vi "Import_Source_Item_Code.vi"(8 "CONTROL Control":enum32{"IMPRORT", "ADD"}(tab), 9 "UPDATE ONLY":bool, 10 "ITEM_DATA":T2, 11 "connection reference":T1) -> ()   [LabVIEW 2015]
uses:
  <vilib>/addons/database/Connection.llb/Conn ObjectReference.ctl
  Controls/ITEM_INFORMATION_CLUSTER.ctl
  <vilib>/addons/database/Connection.llb/Conn Execute.vi
  <vilib>/addons/database/Recordset.llb/Rec Destroy - Connection.vi
  <vilib>/addons/database/_DB Variant To Data/Database Variant To Data.xnode
  <vilib>/addons/database/NI_Database_API.lvlib
  <vilib>/addons/database/Connection.llb/DB Tools Open Connec (String).vi
panel:
  out "UPDATE ONLY 2":bool
  in  "ADD Button":bool
  in  "EXIT_BUTTON":bool
  out "OK":i32
  out "ERROR":i32
  out "Table":string[][](table)
  in  "IMPORT (*.xlsx)":path
  out "TOTAL":i32
  in  "SHEET":i32
  # "ADD ITEM DATA"
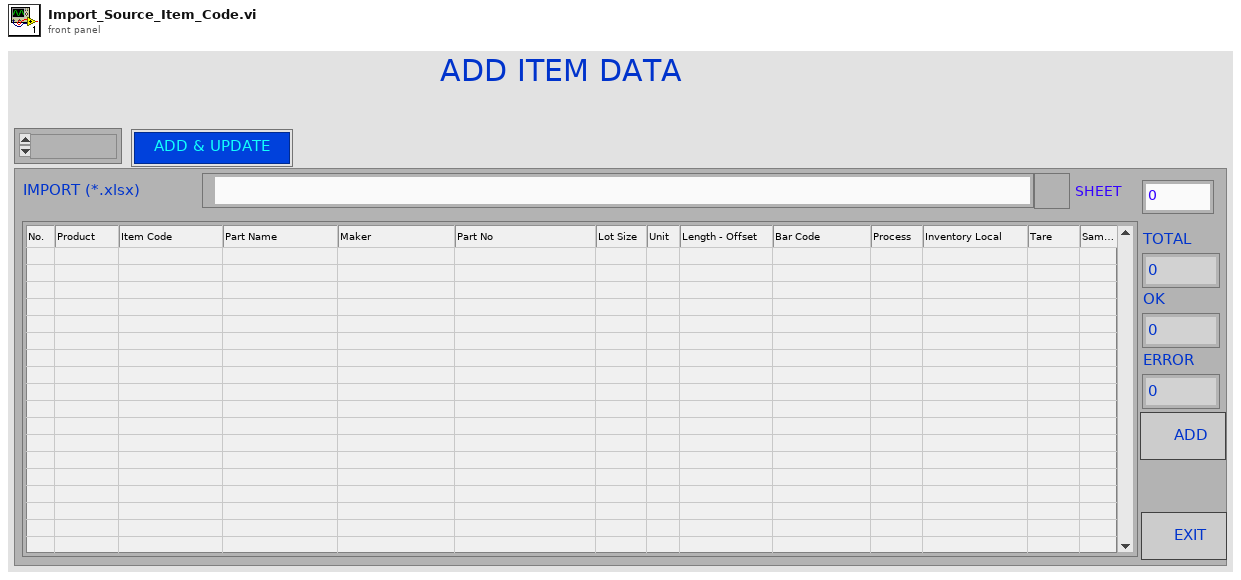
[diagram p1: front panel]
types:
  T1 = typedef "NI_Database_API.lvlib/Conn ObjectReference.ctl" = refnum<k1>
  T2 = cluster{"PRODUCT":string, "ITEM CODE":string, "PART NAME":string, "MAKER":string, "PART NO":string, "LOT SIZE":dbl, "UNIT":string, "LENGTH-OFFSET":string, "BARCODE":string, "PROCESS":string, "INVENTORY LOCAL":string, "TARE":dbl, "SAMPLE":dbl}
  T3 = typedef "ITEM_INFORMATION_CLUSTER.ctl" = cluster{"PRODUCT":string, "ITEM_CODE":string, "PART_NAME":string, "MAKER":string, "PART_NO":string, "LOT_SIZE":dbl, "UNIT":string, "LENGTH-OFFSET":string, "BARCODE":string, "PROCESS":string, "INVENTORY_LOCAL":string, "TARE":dbl, "SAMPLE":dbl}
  T4 = cluster{"PRODUCT":string, "ITEM_CODE":string, "PART_NAME":string, "MAKER":string, "PART_NO":string, "LOT_SIZE":dbl, "UNIT":string, "LENGTH-OFFSET":string, "BARCODE":string, "PROCESS":string, "INVENTORY_LOCAL":string, "TARE":dbl, "SAMPLE":dbl}[]
  T5 = cluster{"start (-1, -1)":cluster{"row":i32, "column":i32}, "end (-1, -1)":cluster{"row":i32, "column":i32}}
  T6 = typedef "NI_Database_API.lvlib/Rec ObjectReference.ctl" = refnum<k1>
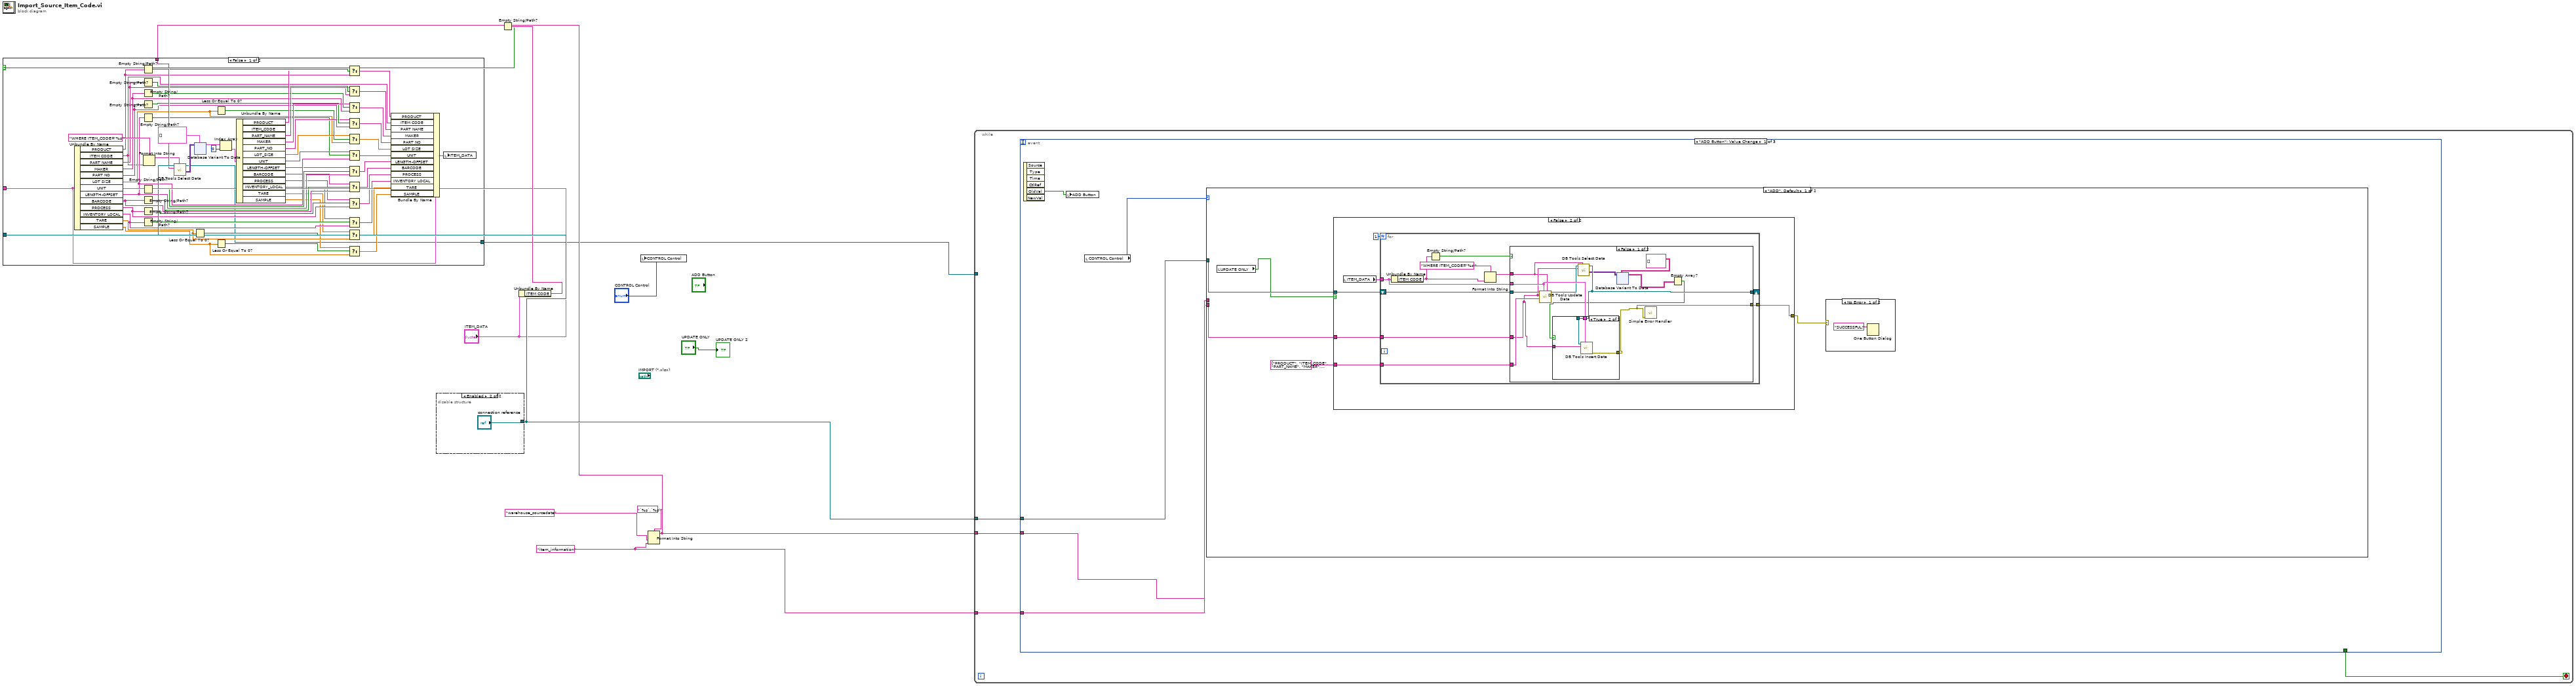
[diagram p0: block diagram]
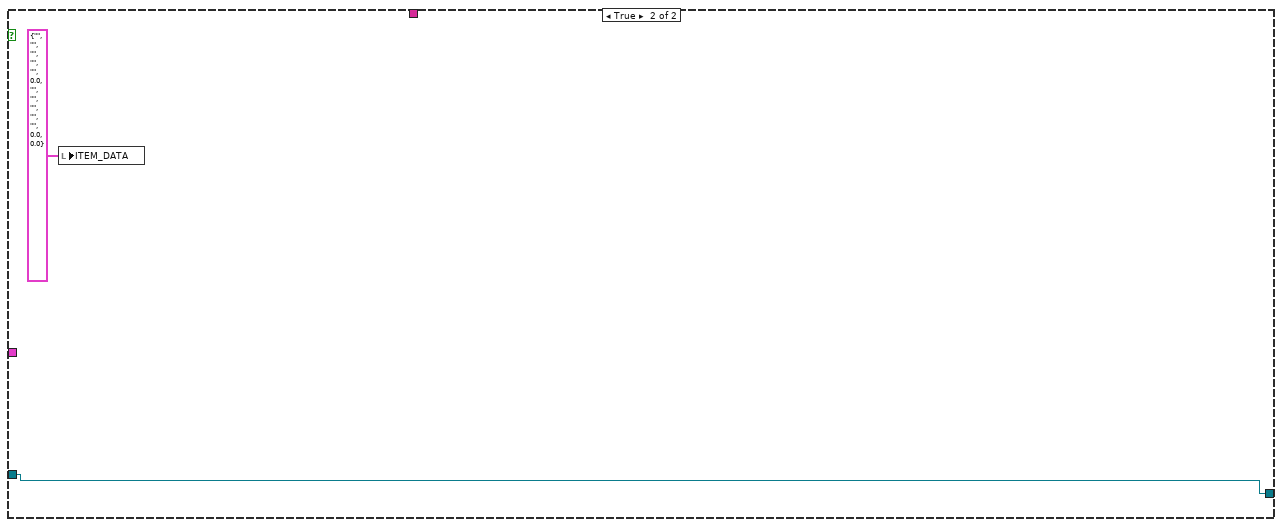
[diagram p2: hidden frame]
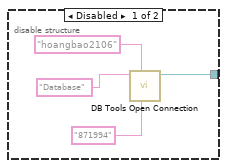
[diagram p3: hidden frame]
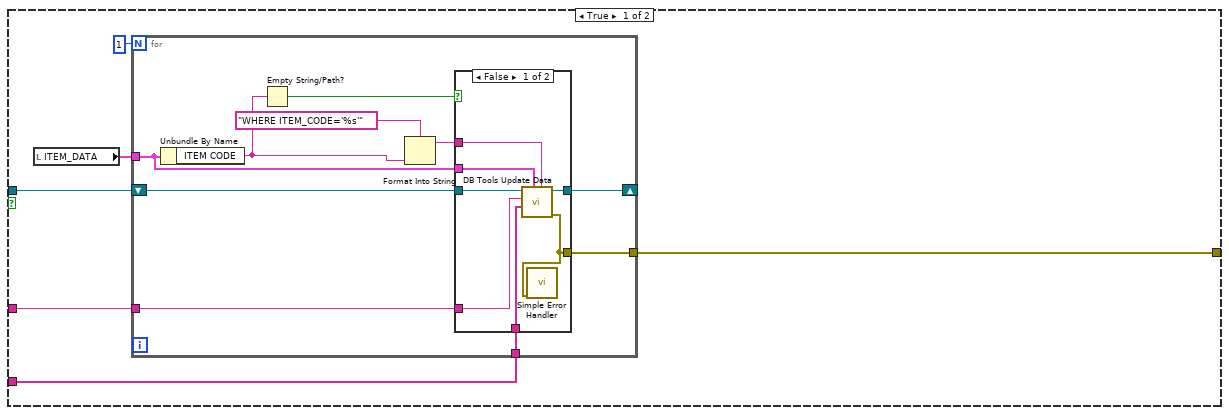
[diagram p5: hidden frame]
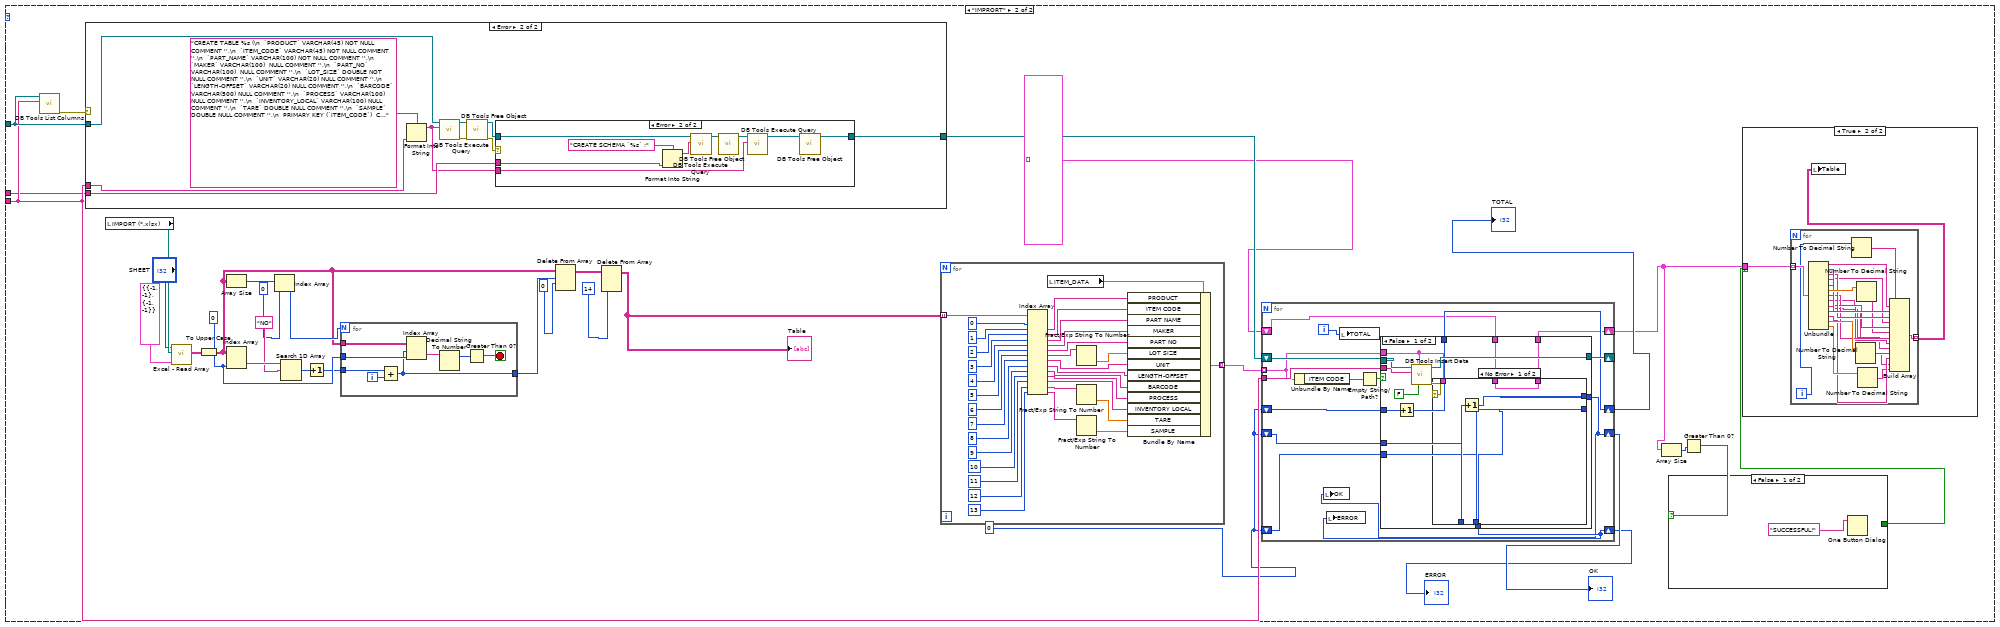
[diagram p9: hidden frame]
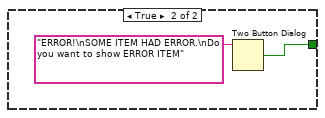
[diagram p11: hidden frame]
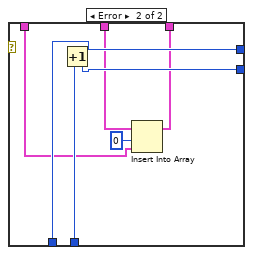
[diagram p12: hidden frame]
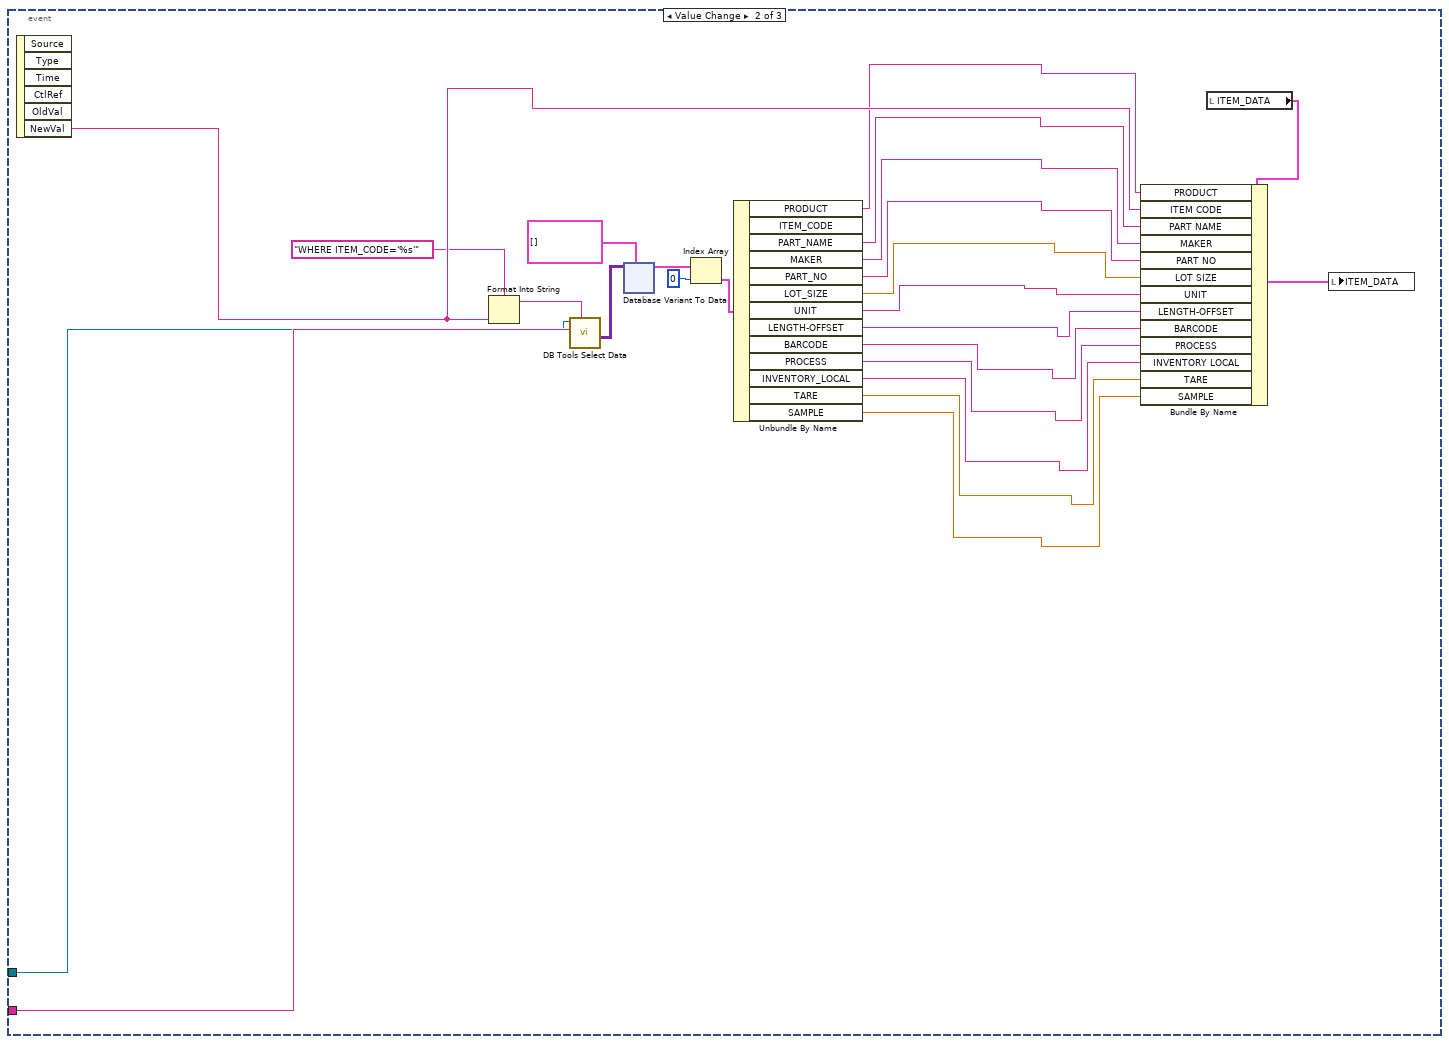
[diagram p16: hidden frame]
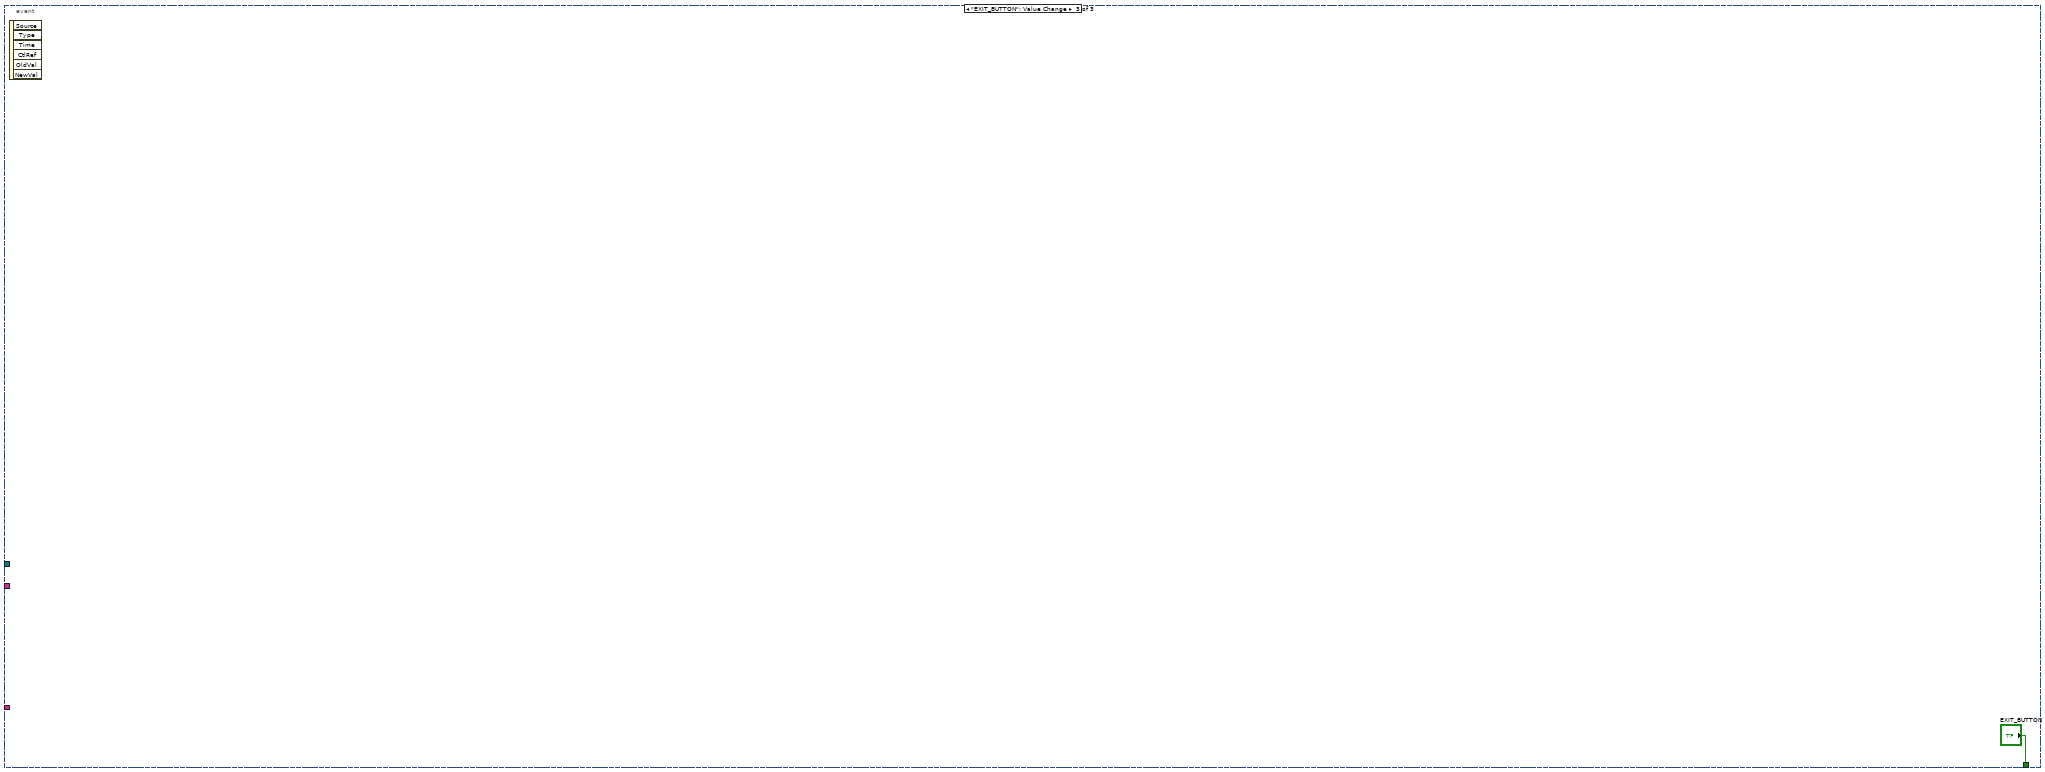
[diagram p17: hidden frame]
diagram:
  w9 = "item_information" ("table")
  n1 = disable-structure shown="Enabled" {
    disable-tunnel: [w12 "connection reference"] -> w6
    frame Disabled {
      n2 = call-poly <vilib>:"DB Tools Open Connection.vi"("password"="871994" ("userID"), "userID"="hoangbao2106", "connection information"="Database" ("userID")) -> ("connection reference"=w12:T1)  [unwired: 5 in, 1 out]
    }
    frame Enabled {
    }
  }
  n3 = Unbundle By Name("ITEM_DATA") -> ("ITEM CODE"=w5:string)
  n4 = Empty String/Path?(string/path=w5) -> (empty?=w4:bool)
  n5 = local write "CONTROL Control"("CONTROL Control") -> ()
  n6 = Format Into String(format string="`%s`.`%s`" ("table"), "warehouse_sourcedata" ("table"), w9) -> (resulting string=w2:string)  [unwired: 2 in, 1 out]
  n7 = case shown="False" w4 {
    tunnel: w6 -> [w77 w491]
    tunnel: "ITEM_DATA" -> [w68 _]
    tunnel: w2 -> [w76 _]
    tunnel: [w17 w491] -> w1
    frame False {
      n8 = Unbundle By Name(w68) -> ("PRODUCT"=w65:string, "ITEM CODE"=w18:string, "PART NAME"=w61:string, "MAKER"=w57:string, "PART NO"=w54:string, "LOT SIZE"=w49:dbl, "UNIT"=w47:string, "LENGTH-OFFSET"=w43:string, "BARCODE"=w37:string, "PROCESS"=w34:string, "INVENTORY LOCAL"=w30:string, "TARE"=w26:dbl, "SAMPLE"=w22:dbl)
      n9 = Empty String/Path?(string/path=w65) -> (empty?=w67:bool)
      n10 = Empty String/Path?(string/path=w61) -> (empty?=w63:bool)
      n11 = Empty String/Path?(string/path=w57) -> (empty?=w59:bool)
      n12 = Empty String/Path?(string/path=w54) -> (empty?=w55:bool)
      n13 = Empty String/Path?(string/path=w47) -> (empty?=w48:bool)
      n14 = Empty String/Path?(string/path=w43) -> (empty?=w44:bool)
      n15 = Empty String/Path?(string/path=w37) -> (empty?=w39:bool)
      n16 = Empty String/Path?(string/path=w34) -> (empty?=w35:bool)
      n17 = Empty String/Path?(string/path=w30) -> (empty?=w31:bool)
      n18 = Format Into String(format string="WHERE ITEM_CODE='%s'", w18) -> (resulting string=w74:string)  [unwired: 2 in, 1 out]
      n19 = call <vilib>:"DB Tools Select Data.vi"("condition"=w74, "table"=w76, "connection reference"=w77) -> ("data"=w73:variant[][], "connection reference out"=w17:T1)  [unwired: 3 in, 1 out]
      n20 = Less Or Equal To 0?(x=w26) -> (x <= 0?=w27:bool)
      n21 = xnode "Database Variant To Data"("database variant"=w73, "type"=T3[] []) -> ("data"=w71:T3[])  [unwired: 1 in, 1 out]
      n22 = Less Or Equal To 0?(x=w49) -> (x <= 0?=w51:bool)
      n23 = Less Or Equal To 0?(x=w22) -> (x <= 0?=w23:bool)
      n24 = Index Array(array=w71, index=0) -> (element=w69:T3)
      n25 = Unbundle By Name(w69) -> ("PRODUCT"=w66:string, "PART_NAME"=w62:string, "MAKER"=w56:string, "PART_NO"=w53:string, "LOT_SIZE"=w50:dbl, "UNIT"=w41:string, "LENGTH-OFFSET"=w42:string, "BARCODE"=w36:string, "PROCESS"=w33:string, "INVENTORY_LOCAL"=w29:string, "TARE"=w25:dbl, "SAMPLE"=w21:dbl)  [unwired: 1 out]
      n26 = Select(t=w66, s=w67, f=w65) -> (s? t:f=w64:string)
      n27 = Select(t=w62, s=w63, f=w61) -> (s? t:f=w60:string)
      n28 = Select(t=w56, s=w59, f=w57) -> (s? t:f=w58:string)
      n29 = Select(t=w53, s=w55, f=w54) -> (s? t:f=w52:string)
      n30 = Select(t=w50, s=w51, f=w49) -> (s? t:f=w45:dbl)
      n31 = Select(t=w41, s=w48, f=w47) -> (s? t:f=w46:string)
      n32 = Select(t=w42, s=w44, f=w43) -> (s? t:f=w40:string)
      n33 = Select(t=w36, s=w39, f=w37) -> (s? t:f=w38:string)
      n34 = Select(t=w33, s=w35, f=w34) -> (s? t:f=w32:string)
      n35 = Select(t=w29, s=w31, f=w30) -> (s? t:f=w28:string)
      n36 = Select(t=w25, s=w27, f=w26) -> (s? t:f=w24:dbl)
      n37 = Select(t=w21, s=w23, f=w22) -> (s? t:f=w20:dbl)
      n38 = Bundle By Name(cluster=w68, "PRODUCT"=w64, "ITEM CODE"=w18, "PART NAME"=w60, "MAKER"=w58, "PART NO"=w52, "LOT SIZE"=w45, "UNIT"=w46, "LENGTH-OFFSET"=w40, "BARCODE"=w38, "PROCESS"=w32, "INVENTORY LOCAL"=w28, "TARE"=w24, "SAMPLE"=w20) -> (w19:T2)
      n39 = local write "ITEM_DATA"(w19) -> ()
    }
    frame True {
      n40 = local write "ITEM_DATA"(T3 {"PRODUCT"="", "ITEM_CODE"="", "PART_NAME"="", "MAKER"="", "PART_NO"="", "LOT_SIZE"=0.0, "UNIT"="", "LENGTH-OFFSET"="", "BARCODE"="", "PROCESS"="", "INVENTORY_LOCAL"="", "TARE"=0.0, "SAMPLE"=0.0} ("ITEM_INFORMATION_Cluster")) -> ()
    }
  }
  n41 = while {
    tunnel: w9 -> [w495]
    tunnel: w2 -> [w494]
    tunnel: w6 -> [w493]
    tunnel: w1 -> [_]
    stop <- w496 stop-if-true
    n42 = event shown="[0] \"ADD Button\": Value Change" {
      selector: _ -> [_ _ _]
      dyn-events: _ -> [_ _ _]
      timeout: _ -> [_ _ _]
      tunnel: [_ _ "EXIT_BUTTON"] -> w496
      tunnel: w495 -> [w501 _ _]
      tunnel: w494 -> [w500 w775 _]
      tunnel: w493 -> [w497 w774 _]
      event "ADD Button": Value Change {
        n43 = event-data() -> ("OldVal"=w498:bool)  [unwired: 1 in, 5 out]
        n44 = local write "ADD Button"(w498) -> ()
        n45 = local read "CONTROL Control"() -> (w499:enum32{"IMPRORT", "ADD"})
        n46 = case shown="\"ADD\", Default" w499 {
          tunnel: w497 -> [w505 w629]
          tunnel: w500 -> [w506 w620]
          tunnel: w501 -> [_ w619]
          frame "ADD", Default {
            n47 = local read "UPDATE ONLY"() -> (w504:bool)
            n48 = case shown="False" w504 {
              tunnel: w506 -> [w513 w537]
              tunnel: w505 -> [w511 w535]
              tunnel: string[] ["PRODUCT", "ITEM_CODE", "PART_NAME", "MAKER", "PART_NO", "LOT_SIZE", "UNIT", "`LENGTH-OFFSET`", "BARCODE", "PROCESS", "INVENTORY_LOCAL", "TARE", "SAMPLE"] ("columns") -> [w509 w533]
              tunnel: [w508 w532] -> w502
              frame True {
                n49 = local read "ITEM_DATA"() -> (w512:T2)
                n50 = for {
                  N: 1 -> [_]
                  tunnel: w513 -> [w521]
                  shift-right: [w522] -> _
                  shift-left: w511 -> [w523]
                  tunnel: w512 -> [w519]
                  tunnel: w509 -> [w515]
                  tunnel: [w514] -> w508
                  n51 = Unbundle By Name(w519) -> ("ITEM CODE"=w517:string)
                  n52 = Empty String/Path?(string/path=w517) -> (empty?=w520:bool)
                  n53 = Format Into String(format string="WHERE ITEM_CODE='%s'" ("condition"), w517) -> (resulting string=w516:string)  [unwired: 2 in, 1 out]
                  n54 = case shown="False" w520 {
                    tunnel: w523 -> [w530 w531]
                    tunnel: [w529 w531] -> w522
                    tunnel: w521 -> [w528 _]
                    tunnel: w519 -> [w527 _]
                    tunnel: w516 -> [w526 _]
                    tunnel: w515 -> [w525 _]
                    tunnel: [w524 _] -> w514
                    frame False {
                      n55 = call <vilib>:"DB Tools Update Data.vi"("condition"=w526, "data"=w527, "columns"=w525, "table"=w528, "connection reference"=w530) -> ("error out"=w524:errorcluster, "connection reference out"=w529:T1)  [unwired: 5 in]
                      n56 = call <vilib>:"Simple Error Handler.vi"("error in (no error)"=w524) -> ()  [unwired: 4 in, 5 out]
                    }
                    frame True {
                    }
                  }
                }
              }
              frame False {
                n57 = local read "ITEM_DATA"() -> (w536:T2)
                n58 = for {
                  N: 1 -> [_]
                  tunnel: w537 -> [w545]
                  shift-right: [w546] -> _
                  shift-left: w535 -> [w547]
                  tunnel: w536 -> [w543]
                  tunnel: w533 -> [w539]
                  tunnel: [w538] -> w532
                  n59 = Unbundle By Name(w543) -> ("ITEM CODE"=w541:string)
                  n60 = Empty String/Path?(string/path=w541) -> (empty?=w544:bool)
                  n61 = Format Into String(format string="WHERE ITEM_CODE='%s'" ("condition"), w541) -> (resulting string=w540:string)  [unwired: 2 in, 1 out]
                  n62 = case shown="False" w544 {
                    tunnel: w547 -> [w559 w608]
                    tunnel: [w552 w608] -> w546
                    tunnel: w545 -> [w554 _]
                    tunnel: w543 -> [w557 _]
                    tunnel: w540 -> [w553 _]
                    tunnel: w539 -> [w558 _]
                    tunnel: [w556 _] -> w538
                    frame False {
                      n63 = call <vilib>:"DB Tools Update Data.vi"("condition"=w553, "data"=w557, "columns"=w558, "table"=w554, "connection reference"=w559) -> ("connection reference out"=w555:T1)  [unwired: 5 in, 1 out]
                      n64 = call <vilib>:"DB Tools Select Data.vi"("condition"=w553, "table"=w554, "connection reference"=w555) -> ("data"=w551:variant[][], "connection reference out"=w552:T1)  [unwired: 3 in, 1 out]
                      n65 = xnode "Database Variant To Data"("database variant"=w551, "type"=string[][] []) -> ("data"=w549:string[][])  [unwired: 1 in, 1 out]
                      n66 = Empty Array?(array=w549) -> (empty?=w548:bool)
                      n67 = case shown="True" w548 {
                        tunnel: w552 -> [_ w607]
                        tunnel: w554 -> [_ w606]
                        tunnel: w557 -> [_ w605]
                        tunnel: [_ w604] -> w556
                        frame False {
                        }
                        frame True {
                          n68 = call <vilib>:"DB Tools Insert Data.vi"("data"=w605, "table"=w606, "connection reference"=w607) -> ("error out"=w604:errorcluster)  [unwired: 7 in, 1 out]
                        }
                      }
                      n69 = call <vilib>:"Simple Error Handler.vi"("error in (no error)"=w556) -> ()  [unwired: 4 in, 5 out]
                    }
                    frame True {
                    }
                  }
                }
              }
            }
            n70 = case shown="No Error" w502 {
              frame No Error {
                n71 = One Button Dialog(message="SUCCESSFUL!") -> ()  [unwired: 1 in, 1 out]
              }
              frame Error {
              }
            }
          }
          frame "IMPRORT" {
            w617 = 0
            w637 = 0 ("disabled index (col)")
            n72 = call <vilib>:"DB Tools List Columns.vi"("table"=w620, "connection reference"=w629) -> ("error out"=w628:errorcluster)  [unwired: 2 in, 3 out]
            n73 = case shown="Error" w628 {
              tunnel: w629 -> [w745 w755]
              tunnel: [w745 w751] -> w623
              tunnel: w620 -> [_ w748]
              tunnel: w619 -> [_ w749]
              frame No Error {
              }
              frame Error {
                n74 = Format Into String(format string="CREATE TABLE %s (\n  `PRODUCT` VARCHAR(45) NOT NULL COMMENT '',\n  `ITEM_CODE` VARCHAR(45) NOT NULL COMMENT '',\n  `PART_NAME` VARCHAR(100) NOT NULL COMMENT '',\n  `MAKER` VARCHAR(100)  NULL COMMENT '',\n  `PART_NO` VARCHAR(100)  NULL COMMENT '',\n  `LOT_SIZE` DOUBLE NOT NULL COMMENT '',\n  `UNIT` VARCHAR(20) NULL COMMENT '',\n  `LENGTH-OFFSET` VARCHAR(20) NULL COMMENT '',\n  `BARCODE` VARCHAR(500) NULL COMMENT '',\n  `PROCESS` VARCHAR(100) NULL COMMENT '',\n  `INVENTORY_LOCAL` VARCHAR(100) NULL COMMENT '',\n  `TARE` DOUBLE NULL COMMENT '',\n  `SAMPLE` DOUBLE NULL COMMENT '',\n  PRIMARY KEY (`ITEM_CODE`)  COMMENT '')" ("SQL query"), w748) -> (resulting string=w746:string)  [unwired: 2 in, 1 out]
                n75 = call-poly <vilib>:"DB Tools Execute Query.vi"("SQL query"=w746, "connection reference"=w755) -> ("error out"=w754:errorcluster, "recordset reference"=w753:T6)  [unwired: 6 in]
                n76 = call-poly <vilib>:"DB Tools Free Object.vi"("error in (no error)"=w754, "recordset reference"=w753) -> ("error out"=w750:errorcluster, "connection reference"=w752:T1)  [unwired: 8 in]
                n77 = case shown="Error" w750 {
                  tunnel: w752 -> [w756 w765]
                  tunnel: [w756 w761] -> w751
                  tunnel: w749 -> [_ w760]
                  tunnel: w746 -> [_ w757]
                  frame No Error {
                  }
                  frame Error {
                    n78 = Format Into String(format string="CREATE SCHEMA `%s` ;" ("SQL query"), w760) -> (resulting string=w758:string)  [unwired: 2 in, 1 out]
                    n79 = call-poly <vilib>:"DB Tools Execute Query.vi"("SQL query"=w758, "connection reference"=w765) -> ("recordset reference"=w764:T6)  [unwired: 6 in, 1 out]
                    n80 = call-poly <vilib>:"DB Tools Free Object.vi"("recordset reference"=w764) -> ("connection reference"=w763:T1)  [unwired: 9 in, 1 out]
                    n81 = call-poly <vilib>:"DB Tools Execute Query.vi"("SQL query"=w757, "connection reference"=w763) -> ("recordset reference"=w762:T6)  [unwired: 6 in, 1 out]
                    n82 = call-poly <vilib>:"DB Tools Free Object.vi"("recordset reference"=w762) -> ("connection reference"=w761:T1)  [unwired: 9 in, 1 out]
                  }
                }
              }
            }
            n83 = local read "IMPORT (*.xlsx)"() -> (w641:path)
            n84 = call "Excel - Read Array.vi"("Cluster"=T5 {"start (-1, -1)"={"row"=-1, "column"=-1}, "end (-1, -1)"={"row"=-1, "column"=-1}}, "Path"=w641, "worksheet index (0)"="SHEET") -> ("Element 1"=w622:string[][])  [unwired: 5 in, 1 out]
            n85 = To Upper Case(1:w622) -> (0:w621:string[][])
            n86 = Array Size(array=w621) -> (size(s)=w632:i32[])
            n87 = Index Array(array=w621, index (col)=w637) -> (element=w639:string[])  [unwired: 1 in]
            n88 = Index Array(array=w632, index=0) -> (element=w630:i32)
            n89 = Search 1D Array(1D array=w639, element="NO") -> (index of element=w636:i32)  [unwired: 1 in]
            n90 = Increment(x=w636) -> (x+1=w635:i32)
            n91 = for {
              N: w630 -> [_]
              tunnel: w635 -> [w770]
              tunnel: w621 -> [w773]
              tunnel: w637 -> [w772]
              tunnel: [w766] -> w633
              i -> [w771]
              stop <- w767 stop-if-true
              n92 = Add(x=w770, y=w771) -> (x+y=w766:i32)
              n93 = Index Array(array=w773, index (row)=w766, index (col)=w772) -> (element=w769:string)
              n94 = Decimal String To Number(string=w769) -> (offset past number=w768:i32)  [unwired: 2 in, 1 out]
              n95 = Greater Than 0?(x=w768) -> (x > 0?=w767:bool)
            }
            n96 = Delete From Array(array=w621, length=w633, index (row)=0) -> (array with subset deleted=w627:string[][])  [unwired: 1 in, 1 out]
            n97 = Delete From Array(array=w627, index (col)=14 ("disabled index (col)")) -> (array with subset deleted=w625:string[][])  [unwired: 2 in, 1 out]
            "Table" <- w625
            n98 = for {
              tunnel: w625 -> [w744] mode=indexing
              tunnel: [w713] -> w624 mode=indexing
              n99 = Index Array(array=w744, index #1=0 ("index"), index #2=1 ("index"), index #3=2 ("index"), index #4=3 ("index"), index #5=4 ("index"), index #6=5 ("index"), index #7=6 ("index"), index #8=7 ("index"), index #9=8 ("index"), index #10=9 ("index"), index #11=10 ("index"), index #12=11 ("index"), index #13=12 ("index"), index #14=13 ("index")) -> (element #2=w714:string, element #3=w715:string, element #4=w716:string, element #5=w717:string, element #6=w718:string, element #7=w720:string, element #8=w721:string, element #9=w722:string, element #10=w723:string, element #11=w724:string, element #12=w725:string, element #13=w727:string, element #14=w728:string)  [unwired: 1 out]
              n100 = local read "ITEM_DATA"() -> (w712:T2)
              n101 = Fract/Exp String To Number(string=w720) -> (number=w719:dbl)  [unwired: 3 in, 1 out]
              n102 = Fract/Exp String To Number(string=w727) -> (number=w726:dbl)  [unwired: 3 in, 1 out]
              n103 = Fract/Exp String To Number(string=w728) -> (number=w729:dbl)  [unwired: 3 in, 1 out]
              n104 = Bundle By Name(cluster=w712, "PRODUCT"=w714, "ITEM CODE"=w715, "PART NAME"=w716, "MAKER"=w717, "PART NO"=w718, "LOT SIZE"=w719, "UNIT"=w721, "LENGTH-OFFSET"=w722, "BARCODE"=w723, "PROCESS"=w724, "INVENTORY LOCAL"=w725, "TARE"=w726, "SAMPLE"=w729) -> (w713:T2)
            }
            n105 = for {
              tunnel: w620 -> [w679]
              shift-right: [w680] -> _
              shift-left: w623 -> [w681]
              tunnel: w624 -> [w676] mode=indexing
              shift-right: [w668] -> w614
              shift-left: w617 -> [w673]
              shift-right: [w667] -> w615
              shift-left: w617 -> [w674]
              shift-right: [w672] -> w616
              shift-left: w617 -> [w675]
              shift-right: [w670] -> w612
              shift-left: T4 [] -> [w671]
              i -> [w669]
              n106 = Unbundle By Name(w676) -> ("ITEM CODE"=w678:string)
              n107 = local write "TOTAL"(w669) -> ()
              n108 = Empty String/Path?(string/path=w678) -> (empty?=w677:bool)
              n109 = case shown="False" w677 {
                tunnel: w681 -> [w695 w711]
                tunnel: [w694 w711] -> w680
                tunnel: w679 -> [w692 _]
                tunnel: w676 -> [w684 _]
                tunnel: w675 -> [w690 w710]
                tunnel: [w689 w710] -> w672
                tunnel: w674 -> [w688 w709]
                tunnel: w673 -> [w687 w708]
                tunnel: [w686 w709] -> w667
                tunnel: [w685 w708] -> w668
                tunnel: w671 -> [w683 w707]
                tunnel: [w682 w707] -> w670
                frame False {
                  n110 = Increment(x=w690) -> (x+1=w689:i32)
                  n111 = call <vilib>:"DB Tools Insert Data.vi"("flatten cluster? (F)"=FALSE, "data"=w684, "table"=w692, "connection reference"=w695) -> ("error out"=w691:errorcluster, "connection reference out"=w694:T1)  [unwired: 6 in]
                  n112 = case shown="No Error" w691 {
                    tunnel: w688 -> [w699 w705]
                    tunnel: w687 -> [w697 w706]
                    tunnel: [w698 w705] -> w686
                    tunnel: [w697 w704] -> w685
                    tunnel: w684 -> [_ w701]
                    tunnel: w683 -> [w696 w703]
                    tunnel: [w696 w700] -> w682
                    frame No Error {
                      n113 = Increment(x=w699) -> (x+1=w698:i32)
                    }
                    frame Error {
                      n114 = Increment(x=w706) -> (x+1=w704:i32)
                      n115 = Insert Into Array(array=w703, index=0, new element=w701) -> (w700:T4)
                    }
                  }
                }
                frame True {
                }
              }
              n116 = local write "OK"(w667) -> ()
              n117 = local write "ERROR"(w668) -> ()
            }
            "TOTAL" <- w616
            "OK" <- w615
            "ERROR" <- w614
            n118 = Array Size(array=w612) -> (size(s)=w611:i32)
            n119 = Greater Than 0?(x=w611) -> (x > 0?=w610:bool)
            n120 = case shown="False" w610 {
              tunnel: [_ w665] -> w609
              frame False {
                n121 = One Button Dialog(message="SUCCESSFUL!") -> ()  [unwired: 1 in, 1 out]
              }
              frame True {
                n122 = Two Button Dialog(message="ERROR!\nSOME ITEM HAD ERROR.\nDo you want to show ERROR ITEM") -> (T button?=w665:bool)  [unwired: 2 in]
              }
            }
            n123 = case shown="True" w609 {
              tunnel: w612 -> [_ w642]
              frame False {
              }
              frame True {
                n124 = for {
                  tunnel: w642 -> [w663] mode=indexing
                  tunnel: [w646] -> w643 mode=indexing
                  i -> [w645]
                  n125 = Unbundle(w663) -> ("PRODUCT"=w659:string, "ITEM_CODE"=w658:string, "PART_NAME"=w657:string, "MAKER"=w656:string, "PART_NO"=w655:string, "LOT_SIZE"=w662:dbl, "UNIT"=w653:string, "LENGTH-OFFSET"=w652:string, "BARCODE"=w651:string, "PROCESS"=w650:string, "INVENTORY_LOCAL"=w649:string, "TARE"=w661:dbl, "SAMPLE"=w660:dbl)
                  n126 = Number To Decimal String(number=w645) -> (decimal integer string=w644:string)  [unwired: 1 in]
                  n127 = Number To Decimal String(number=w661) -> (decimal integer string=w648:string)  [unwired: 1 in]
                  n128 = Number To Decimal String(number=w662) -> (decimal integer string=w654:string)  [unwired: 1 in]
                  n129 = Number To Decimal String(number=w660) -> (decimal integer string=w647:string)  [unwired: 1 in]
                  n130 = Build Array(w644, w659, w658, w657, w656, w655, w654, w653, w652, w651, w650, w649, w648, w647) -> (w646:string[])
                }
                n131 = local write "Table"(w643) -> ()
              }
            }
          }
        }
      }
      event "ITEM_DATA.ITEM CODE": Value Change {
        n132 = event-data() -> ("NewVal"=w797:string)  [unwired: 1 in, 5 out]
        n133 = Format Into String(format string="WHERE ITEM_CODE='%s'", w797) -> (resulting string=w795:string)  [unwired: 2 in, 1 out]
        n134 = call <vilib>:"DB Tools Select Data.vi"("condition"=w795, "table"=w775, "connection reference"=w774) -> ("data"=w794:variant[][])  [unwired: 3 in, 2 out]
        n135 = xnode "Database Variant To Data"("database variant"=w794, "type"=T3[] []) -> ("data"=w792:T3[])  [unwired: 1 in, 1 out]
        n136 = Index Array(array=w792, index=0) -> (element=w790:T3)
        n137 = Unbundle By Name(w790) -> ("PRODUCT"=w789:string, "PART_NAME"=w788:string, "MAKER"=w787:string, "PART_NO"=w786:string, "LOT_SIZE"=w785:dbl, "UNIT"=w784:string, "LENGTH-OFFSET"=w783:string, "BARCODE"=w782:string, "PROCESS"=w781:string, "INVENTORY_LOCAL"=w780:string, "TARE"=w779:dbl, "SAMPLE"=w778:dbl)  [unwired: 1 out]
        n138 = local read "ITEM_DATA"() -> (w776:T2)
        n139 = Bundle By Name(cluster=w776, "PRODUCT"=w789, "ITEM CODE"=w797, "PART NAME"=w788, "MAKER"=w787, "PART NO"=w786, "LOT SIZE"=w785, "UNIT"=w784, "LENGTH-OFFSET"=w783, "BARCODE"=w782, "PROCESS"=w781, "INVENTORY LOCAL"=w780, "TARE"=w779, "SAMPLE"=w778) -> (w777:T2)
        n140 = local write "ITEM_DATA"(w777) -> ()
      }
      event "EXIT_BUTTON": Value Change {
        n141 = event-data() -> ()  [unwired: 1 in, 6 out]
      }
    }
  }
  "UPDATE ONLY 2" <- "UPDATE ONLY"
